vi "okCFrontPanel Update Wire Ins.vi"(8 "Error In":errorcluster, 11 "okCFrontPanel Refnum":refnum<k24>) -> (0 "Error Out":errorcluster, 3 "okCFrontPanel Refnum":refnum<k24>)   [LabVIEW 2019, in "okFrontPanelC#Wrapper.lvlib"]
uses:
  okFrontPanelC#Wrapper.lvlib
  C:/UCLA Thinkpad Google Drive/LabVIEW 2019 SP1/builds/SS2 Live Distribution/Opal Kelly/C# Wrapper/libFrontPanel-csharp.dll
  libFrontPanel-csharp.dll
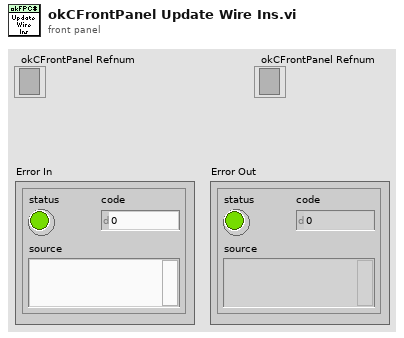
[diagram p1: front panel]
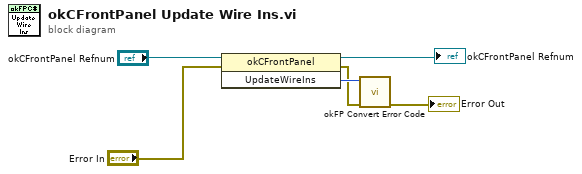
[diagram p0: block diagram]
diagram:
  n1 = invoke class="okCFrontPanel" method="UpdateWireIns"(reference="okCFrontPanel Refnum", error in="Error In") -> (reference out=→"okCFrontPanel Refnum":refnum<k24>, error out=w2:errorcluster, "UpdateWireIns"=w3:i32)  [unwired: 1 in]
  n2 = call "okFP Convert Error Code.vi"("error in (no error)"=w2, "okFP Error Code"=w3) -> ("error out"=→"Error Out":errorcluster)  [unwired: 9 in]
